vi "TestBench.vi"() -> ()   [LabVIEW 2015]
uses:
  SPWM/Signal.ctl
  SPWM/SPWM.lvlib
  SPWMInterface/SPWMInterface.lvlib
  <vilib>/measure/NI_MABase.lvlib
panel:
  out "Numeric":i32
  out "Waveform Graph":dbl[][](graph)
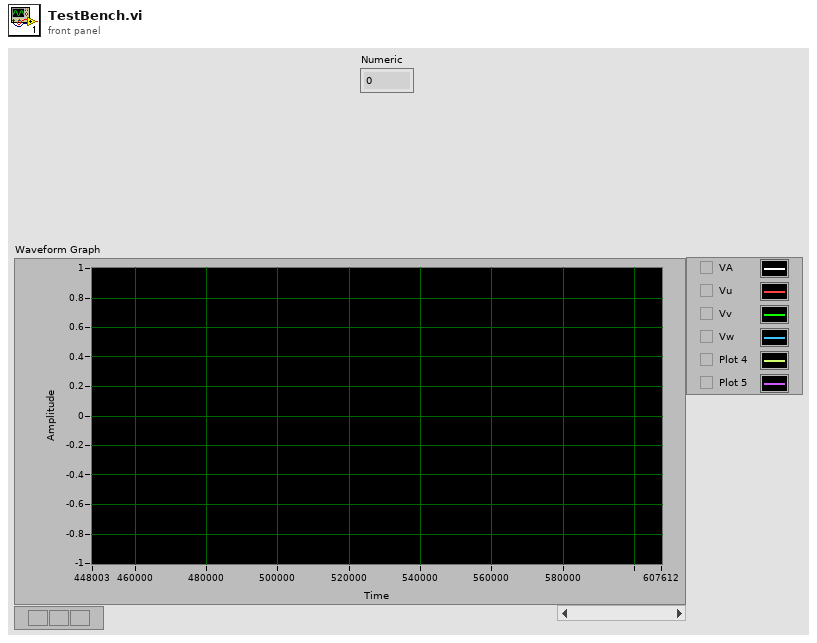
[diagram p1: front panel]
types:
  T1 = typedef "SPWM.lvlib/SwitchConfig.ctl" = cluster{"FreqCarrier":u32, "DeadtimeTicks":u8, "TriangleInc":fxp<+/-,32,4>}
  T2 = typedef "SPWM.lvlib/Signal.ctl" = cluster{"A":fxp<+/-,32,4>, "B":fxp<+/-,32,4>, "C":fxp<+/-,32,4>}
  T3 = typedef "SPWM.lvlib/SwitchPositions.ctl" = cluster{"UTop":bool, "UBottom":bool, "VTop":bool, "VBottom":bool, "WTop":bool, "WBottom":bool}
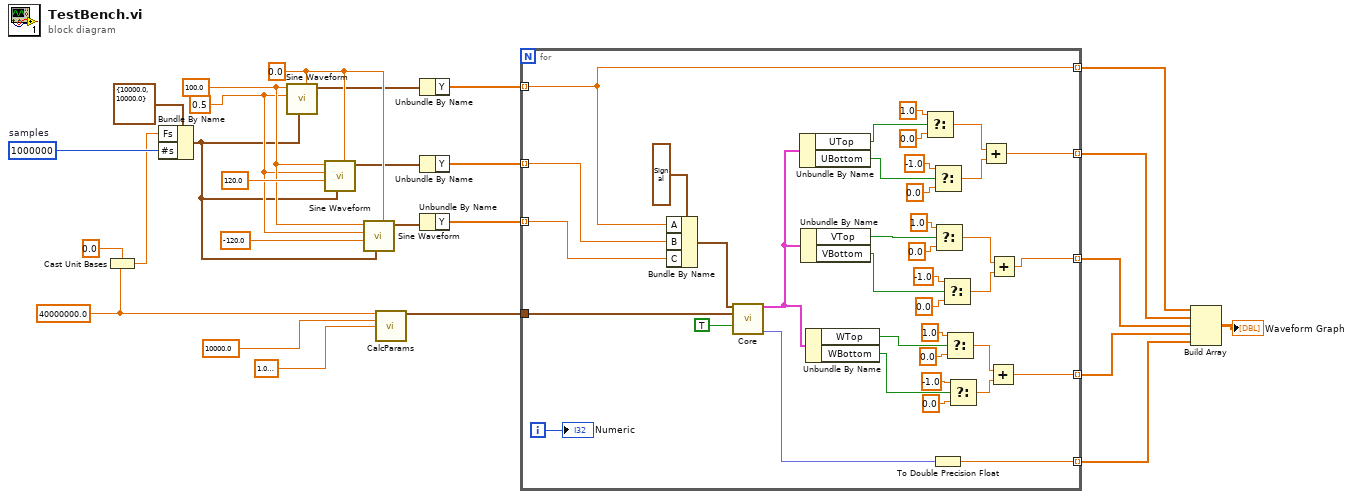
[diagram p0: block diagram]
diagram:
  w8 = dbl[unit] 40000000.0 ("ClkRate")
  w13 = 1000000  # samples
  w24 = 0.0 ("offset")
  w22 = 0.5 ("amplitude")
  w23 = 100.0 ("frequency")
  n1 = Cast Unit Bases(0:w8, 1:0.0 ("unit (none)")) -> (2:w7:dbl)
  n2 = Bundle By Name(cluster=cluster{"Fs":dbl, "#s":dbl} {"Fs"=10000.0, "#s"=10000.0} ("sampling info"), "Fs"=w7, "#s"=w13) -> (w12:cluster{"Fs":dbl, "#s":dbl})
  n3 = call <vilib>:"Sine Waveform.vi"("offset"=w24, "sampling info"=w12, "amplitude"=w22, "frequency"=w23) -> ("signal out"=w20:waveform(dbl))  [unwired: 6 in, 1 out]
  n4 = call <vilib>:"Sine Waveform.vi"("offset"=w24, "sampling info"=w12, "phase"=120.0, "amplitude"=w22, "frequency"=w23) -> ("signal out"=w19:waveform(dbl))  [unwired: 5 in, 1 out]
  n5 = call <vilib>:"Sine Waveform.vi"("offset"=w24, "sampling info"=w12, "phase"=-120.0, "amplitude"=w22, "frequency"=w23) -> ("signal out"=w18:waveform(dbl))  [unwired: 5 in, 1 out]
  n6 = call "CalcParams.vi"("ClkRate"=w8, "fc"=dbl[unit] 10000.0, "Deadtime"=dbl[unit] 1.0000000000000001e-07) -> ("Parameters"=w26:T1)  [unwired: 12 in]
  n7 = Unbundle By Name(w20) -> ("Y"=w17:dbl[])
  n8 = Unbundle By Name(w19) -> ("Y"=w16:dbl[])
  n9 = Unbundle By Name(w18) -> ("Y"=w15:dbl[])
  n10 = for {
    tunnel: w26 -> [w63]
    tunnel: w17 -> [w41] mode=indexing
    tunnel: w16 -> [w40] mode=indexing
    tunnel: w15 -> [w61] mode=indexing
    tunnel: [w58] -> w4 mode=indexing
    tunnel: [w41] -> w3 mode=indexing
    tunnel: [w42] -> w2 mode=indexing
    tunnel: [w29] -> w1 mode=indexing
    tunnel: [w30] -> w5 mode=indexing
    i -> [w57]
    n11 = Bundle By Name(cluster=T2 {"A"=0.0, "B"=0.0, "C"=0.0} ("sine waves"), "A"=w41, "B"=w40, "C"=w61) -> (w60:T2)
    n12 = call "Core.vi"("Signal"=w60, "SwitchConfig"=w63, "enable"=TRUE) -> ("SwitchPositions"=w39:T3, "TriangleWave"=w59:fxp<+/-,32,4>)  [unwired: 11 in]
    n13 = Unbundle By Name(w39) -> ("UTop"=w28:bool, "UBottom"=w27:bool)
    n14 = Unbundle By Name(w39) -> ("VTop"=w44:bool, "VBottom"=w43:bool)
    n15 = Unbundle By Name(w39) -> ("WTop"=w32:bool, "WBottom"=w31:bool)
    n16 = Select(t=1.0, s=w28, f=0.0) -> (s? t:f=w52:dbl)
    n17 = Select(t=-1.0, s=w27, f=0.0) -> (s? t:f=w51:dbl)
    n18 = To Double Precision Float(number=w59) -> (double precision float=w58:dbl)
    n19 = Select(t=1.0, s=w44, f=0.0) -> (s? t:f=w46:dbl)
    n20 = Select(t=-1.0, s=w43, f=0.0) -> (s? t:f=w45:dbl)
    n21 = Select(t=1.0, s=w32, f=0.0) -> (s? t:f=w37:dbl)
    n22 = Select(t=-1.0, s=w31, f=0.0) -> (s? t:f=w38:dbl)
    n23 = Add(x=w52, y=w51) -> (x+y=w42:dbl)
    n24 = Add(x=w37, y=w38) -> (x+y=w30:dbl)
    n25 = Add(x=w46, y=w45) -> (x+y=w29:dbl)
    "Numeric" <- w57
  }
  n26 = Build Array(w3, w2, w1, w5, w4) -> (→"Waveform Graph":dbl[][])
